vi "PriceToDBL.vi"(1 "float string":string) -> (0 "float out":dbl)   [LabVIEW 2024]
uses:
  <vilib>/Utility/error.llb/Trim Whitespace One-Sided.vi
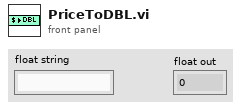
[diagram p1: front panel]
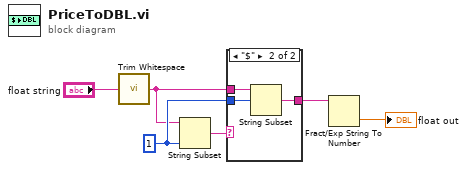
[diagram p0: block diagram]
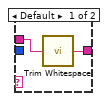
[diagram p2: hidden frame]
diagram:
  w3 = 1 ("length (rest)")
  n1 = call <vilib>:"Trim Whitespace.vi"("string"="float string") -> ("trimmed string"=w1:string)  [unwired: 1 in]
  n2 = String Subset(string=w1, length (rest)=w3) -> (substring=w4:string)  [unwired: 1 in]
  n3 = case shown="\"$\"" w4 {
    tunnel: w1 -> [w7 w11]
    tunnel: w3 -> [_ w10]
    tunnel: [w8 w9] -> w2
    frame Default {
      n4 = call <vilib>:"Trim Whitespace.vi"("string"=w7) -> ("trimmed string"=w8:string)  [unwired: 1 in]
    }
    frame "$" {
      n5 = String Subset(string=w11, offset (0)=w10) -> (substring=w9:string)  [unwired: 1 in]
    }
  }
  n6 = Fract/Exp String To Number(string=w2) -> (number=→"float out":dbl)  [unwired: 3 in, 1 out]
